vi "rsscope_FormatSearchNameTBTOFrameInt32_ReadCallback.vi"(5 "Attribute":T1={"Identifier"="", "Descriptive Name"="", "Data Type"=enum."Integer 32", "Command"="", "Access"=enum."Read/Write", "Range Table"="", "Read Callback"="", "Write Callback"="", "Supported Models"="", "Instrument Options"="", "Index"=0, "OPC Wait"=FALSE, "No Status Check"=FALSE, "Cache Only"=FALSE}, 7 "Repeated Capability":string, 8 "error in (no error)":errorcluster, 11 "VISA resource name":refnum<visa-resource-name>) -> (0 "error out":errorcluster, 2 "Attribute Value I32":i32, 3 "VISA resource name out":refnum<visa-resource-name>)   [LabVIEW 2018]
doc: "This VI sets the attribute value.\n\nThis is a low-level VI that you can use to set the values of instrument-specific properties and inherent IVI properties. If the property represents an instrument state, this VI performs instrument I/O in the following cases:\n\n- State caching is disabled for the entire session or for the particular property.\n\n- State caching is enabled and the currently cached value is invalid or is different than the value you specify. \n\nThis instrument driver contains high-level VIs that set most of the instrument properties. It is best to use the high-level driver VIs as much as possible. They handle order dependencies and multithread locking for you. In addition, they perform status checking only after setting all of the properties. In contrast, when you set multiple properties using the SetAttribute VIs, the VIs check the instrument status after each call.\n\nAlso, when state caching is enabled, the high-level VIs that configure multiple properties perform instrument I/O only for the properties whose value you change. Thus, you can safely call the high-level VIs without the penalty of redundant instrument I/O."
uses:
  rsidr_core.llb/type_Attribute.ctl
  rsidr_core.llb/type_Attribute_Data_Type.ctl
  rsidr_core.llb/type_ReadWriteAccess.ctl
  rsidr_core.llb/rsscope_rsidr_core.lvlib
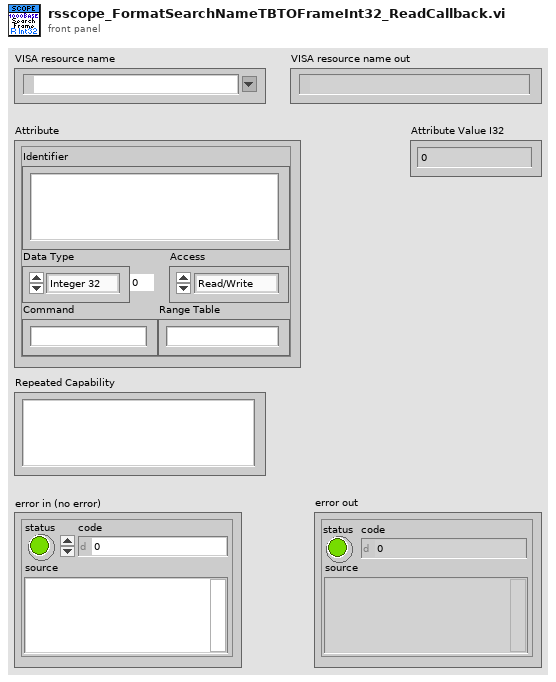
[diagram p1: front panel]
types:
  T1 = typedef "rsscope_rsidr_core.lvlib/type_Attribute.ctl" = cluster{"Identifier":string, "Descriptive Name":string, "Data Type":T2, "Command":string, "Access":T3, "Range Table":string, "Read Callback":string, "Write Callback":string, "Supported Models":string, "Instrument Options":string, "Index":i32, "OPC Wait":bool, "No Status Check":bool, "Cache Only":bool}
  T2 = typedef "rsscope_rsidr_core.lvlib/type_Attribute_Data_Type.ctl" = enum16{"Integer 32", "Double", "String", "Boolean", "None", "Integer 64", "RawString"}
  T3 = typedef "rsscope_rsidr_core.lvlib/type_ReadWriteAccess.ctl" = enum16{"Read Only", "Write Only", "Read/Write"}
  T4 = typedef "rsscope_rsidr_core.lvlib/type_Session_Data.ctl" = cluster{"IDN string":string, "Instrument FW":string, "Instr type":string, "Instr type for err. msg.":string, "Installed Options":string[], "Ignore Error Messages":string, "Logging params":variant, "OPC Timeout":i32, "VISA Timeout":i32, "STB Poll VISA Timeout":i32, "Additional Flags":i32, "Wait Before Read":i32, "Wait Before Write":i32, "Option String Flags":i32, "IO Segment Size":i64, "VISA Access Mode":T5, "Interface Type":T6, "OPC Wait Mode":T7, "Bin Float Number  Format":T8, "Bin Integer Number Format":T9, "Simulate":bool, "VXIcapable":bool, "Duplicate Session":bool, "Add LF to Write":bool, "Logging":bool, "Fast Sweep":bool, "Query Instrument Status":bool, "Check Range":bool, "Check Options":bool}
  T5 = typedef "rsscope_rsidr_core.lvlib/type_VisaAccessMode.ctl" = u16
  T6 = typedef "rsscope_rsidr_core.lvlib/type_InterfaceType.ctl" = enum16{"Unknown", "GPIB", "VXI", "GPIB_VXI", "ASRL", "PXI", "TCPIP", "USB", "SOCKET"}
  T7 = typedef "rsscope_rsidr_core.lvlib/type_OPC_Wait_Mode.ctl" = enum16{"STBpolling", "STBpollingSlow", "STBpollingSuperSlow", "ServiceRequest", "OPCquery"}
  T8 = typedef "rsscope_rsidr_core.lvlib/type_Binary_Float_Number_Format.ctl" = enum16{"Float_4_Bytes_Swapped", "Float_4_Bytes", "Double_8_Bytes_Swapped", "Double_8_Bytes"}
  T9 = typedef "rsscope_rsidr_core.lvlib/type_Binary_Integer_Number_Format.ctl" = enum16{"Int32_4_Bytes_Swapped", "Int32_4 Bytes", "Int16_2_Bytes_Swapped", "Int16_2_Bytes"}
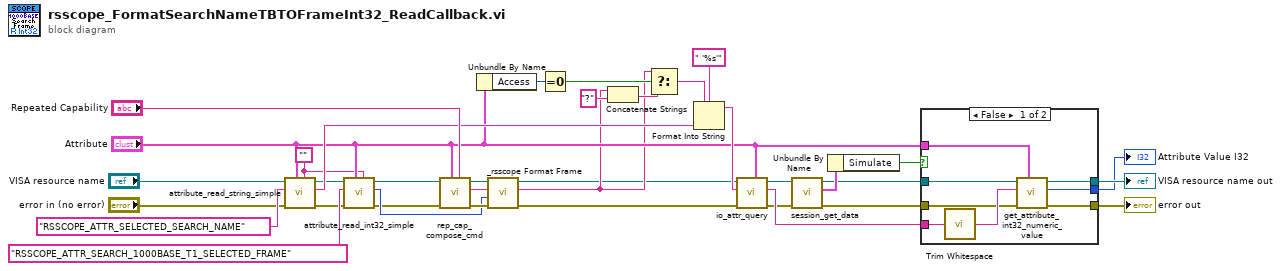
[diagram p0: block diagram]
diagram:
  w10 = "" ("Empty String Constant")
  n1 = call "attribute_read_string_simple.vi"("Repeated Capability"=w10, "Attribute"="Attribute", "error in"="error in (no error)", "Direct Attribute ID (\"\")"="RSSCOPE_ATTR_SELECTED_SEARCH_NAME" ("Direct Attribute ID (\"\")"), "VISA resource name"="VISA resource name") -> ("error out"=w12:errorcluster, "String out"=w31:string, "VISA resource name out"=w13:refnum<visa-resource-name>)  [unwired: 4 in]
  n2 = call "attribute_read_int32_simple.vi"("Repeated Capability"=w10, "Attribute"="Attribute", "error in"=w12, "Direct Attribute ID (\"\")"="RSSCOPE_ATTR_SEARCH_1000BASE_T1_SELECTED_FRAME" ("Direct Attribute ID (\"\")"), "VISA resource name"=w13) -> ("error out"=w1:errorcluster, "Int32 out"=w6:i32, "VISA resource name out"=w2:refnum<visa-resource-name>)  [unwired: 4 in]
  n3 = call "rep_cap_compose_cmd.vi"("Repeated Capability"="Repeated Capability", "Attribute"="Attribute", "error in"=w1, "VISA resource name"=w2) -> ("error out"=w7:errorcluster, "Command out"=w9:string, "VISA resource name out"=w8:refnum<visa-resource-name>)  [unwired: 5 in]
  n4 = Unbundle By Name("Attribute") -> ("Access"=w27:T3)
  n5 = call "_rsscope Format Frame.vi"("error in (no error)"=w7, "Frame (1)"=w6, "Input String"=w9, "VISA resource name"=w8) -> ("error out"=w3:errorcluster, "Output String"=w5:string, "VISA resource name out"=w4:refnum<visa-resource-name>)  [unwired: 5 in]
  n6 = Equal To 0?(x=w27) -> (x = 0?=w26:bool)
  n7 = Concatenate Strings(w5, "?" ("string")) -> (w29:string)
  n8 = Select(t=w5, s=w26, f=w29) -> (s? t:f=w25:string)
  n9 = Format Into String(format string=" '%s'", initial string=w25, w31) -> (resulting string=w30:string)  [unwired: 1 in, 1 out]
  n10 = call "io_attr_query.vi"("Attribute"="Attribute", "error in"=w3, "write buffer"=w30, "VISA resource name"=w4) -> ("error out"=w16:errorcluster, "read buffer"=w17:string, "VISA resource name out"=w15:refnum<visa-resource-name>)  [unwired: 5 in]
  n11 = call "session_get_data.vi"("error in"=w16, "VISA resource name"=w15) -> ("error out"=w23:errorcluster, "Session User Data out"=w24:T4, "VISA resource name out"=w22:refnum<visa-resource-name>)  [unwired: 6 in, 1 out]
  n12 = Unbundle By Name(w24) -> ("Simulate"=w21:bool)
  n13 = case shown="False" w21 {
    tunnel: [w41 w46] -> w19
    tunnel: [w40 w45] -> w20
    tunnel: [w43 _] -> w18
    tunnel: "Attribute" -> [w42 _]
    tunnel: w23 -> [w38 w46]
    tunnel: w22 -> [w37 w45]
    tunnel: w17 -> [w39 _]
    frame False {
      n14 = call <vilib>:"Trim Whitespace.vi"("string"=w39) -> ("trimmed string"=w44:string)  [unwired: 1 in]
      n15 = call "get_attribute_int32_numeric_value.vi"("Attribute"=w42, "error in"=w38, "Cmd Value in"=w44, "VISA resource name"=w37) -> ("error out"=w41:errorcluster, "Int32 value out"=w43:i32, "VISA resource name out"=w40:refnum<visa-resource-name>)  [unwired: 5 in]
    }
    frame True {
    }
  }
  "error out" <- w19
  "VISA resource name out" <- w20
  "Attribute Value I32" <- w18
